vi "PPSU Data.vi"(7 "Write/Read":enum16{"Write", "Read"}(ring)=enum."Read", 11 "PPSU Data":waveform(dbl)[](array[waveform])) -> (3 "Array":waveform(dbl)[](array[waveform]))   [LabVIEW 2022 SP3]
panel:
  out "error out":errorcluster
  in  "error in":errorcluster
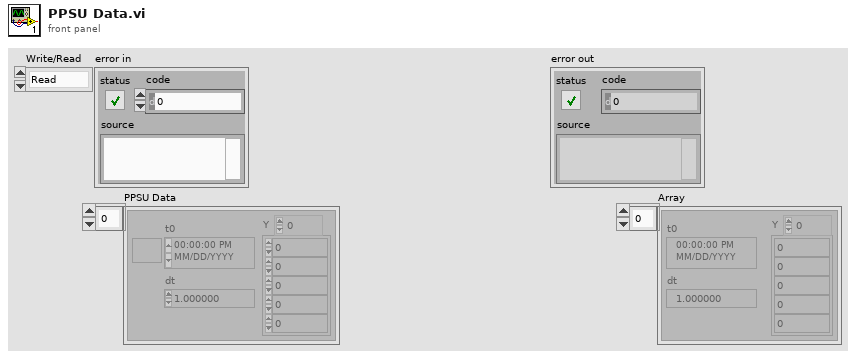
[diagram p1: front panel]
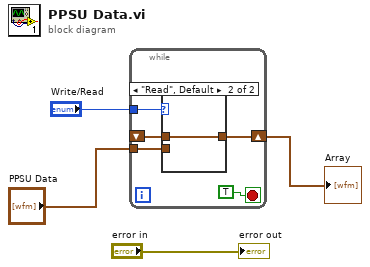
[diagram p0: block diagram]
diagram:
  n1 = while {
    tunnel: "Write/Read" -> [w9]
    tunnel: "PPSU Data" -> [w7]
    shift-right: [w6] -> w1
    shift-left: _ -> [w5]
    stop <- TRUE stop-if-true
    n2 = case shown="\"Read\", Default" w9 {
      tunnel: w7 -> [w10 _]
      tunnel: [w10 w11] -> w6
      tunnel: w5 -> [_ w11]
      frame "Write" {
      }
      frame "Read", Default {
      }
    }
  }
  "Array" <- w1
  "error out" <- "error in"
